vi "get_data.vi"(0 "HGF_SVService.lvclass in":refnum<class "HGF_SVService.lvclass">, 5 "error in (no error)":errorcluster) -> (14 "HGF_SVService.lvclass out":refnum<class "HGF_SVService.lvclass">, 15 "serviceID":i32, 16 "data":string, 17 "quality":i32, 19 "error out":errorcluster)   [LabVIEW 2012, in "HGF_SV.lvlib" / "HGF_SVService.lvclass"]
uses:
  HGF_SVService.lvclass
  HGF_SVService.lvclass/HGF_SVService.ctl
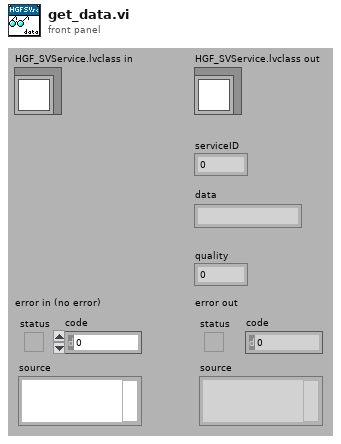
[diagram p1: front panel]
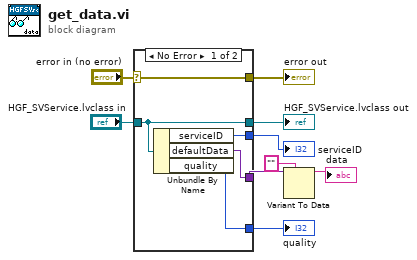
[diagram p0: block diagram]
diagram:
  n1 = case shown="No Error" "error in (no error)" {
    selector: "error in (no error)" -> [w14 w15]
    tunnel: [w14 w15] -> w8
    tunnel: [w13 w16] -> w6
    tunnel: "HGF_SVService.lvclass in" -> [w13 w16]
    tunnel: [w12 _] -> w4
    tunnel: [w11 _] -> w3
    tunnel: [w10 _] -> w5
    frame No Error {
      n2 = Unbundle By Name(w13) -> ("serviceID"=w11:i32, "defaultData"=w12:variant, "quality"=w10:i32)
    }
    frame Error {
    }
  }
  "error out" <- w8
  "HGF_SVService.lvclass out" <- w6
  "serviceID" <- w3
  "quality" <- w5
  n3 = Variant To Data(type="" ("data 2"), Variant=w4) -> (data=→"data":string)  [unwired: 1 in, 1 out]
